vi "程序设置-读取注释.vi"(8 "error in":errorcluster caption="错误输入（无错误）", 11 "程序号":i32) -> (0 "error out":errorcluster, 3 "程序注释":string)   [LabVIEW 2009]
uses:
  <vilib>/Utility/xml.llb/Read From XML File(array).vi
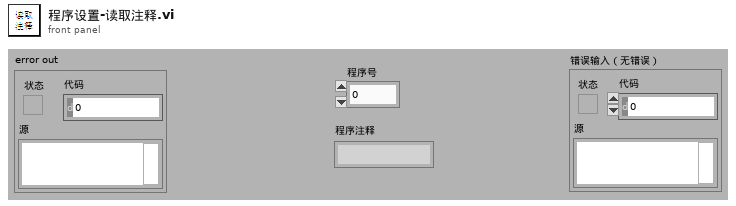
[diagram p1: front panel]
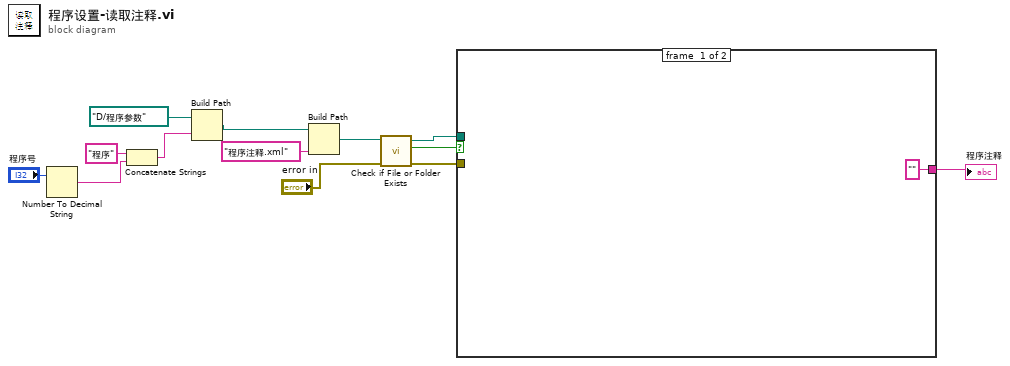
[diagram p0: block diagram]
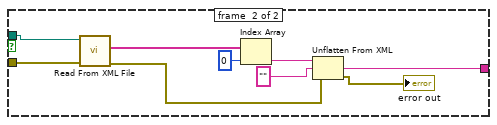
[diagram p2: hidden frame]
diagram:
  n1 = Number To Decimal String(number="程序号") -> (decimal integer string=w8:string)  [unwired: 1 in]
  n2 = Concatenate Strings("程序" ("字符串"), w8) -> (w11:string)
  n3 = Build Path(base path=path "D:/程序参数" ("基路径"), name or relative path=w11) -> (appended path=w7:path)
  n4 = Build Path(base path=w7, name or relative path="程序注释.xml" ("名称或相对路径")) -> (appended path=w6:path)
  n5 = call <vilib>:"Check if File or Folder Exists.vi"("error in (no error)"="error in", "path"=w6) -> ("error out"=w3:errorcluster, "file or folder exists?"=w5:bool, "dup path"=w4:path)  [unwired: 7 in]
  n6 = case shown="真" w5 {
    tunnel: w4 -> [_ w23]
    tunnel: w3 -> [_ w22]
    tunnel: ["" w17] -> w1
    frame #0 {
    }
    frame #1 {
      n7 = call-poly <vilib>:"Read From XML File.vi"("error in (no error)"=w22, "XML File Path"=w23) -> ("error out"=w16:errorcluster, "XML Elements"=w21:string[])  [unwired: 7 in, 1 out]
      n8 = Index Array(array=w21, index=0 ("索引")) -> (element=w19:string)
      n9 = Unflatten From XML(xml string=w19, type="", error in (no error)=w16) -> (value=w17:string, error out=→"error out":errorcluster)
    }
  }
  "程序注释" <- w1
